vi "Booean to T-F string.vi"(4 "Boolean iin":bool) -> (1 "T/F String":string)   [LabVIEW 2009, in "Strings Lib.lvlib"]
doc: "Converts a boolean to 'T' or 'F' String. Used for shortened notation file io."
uses:
  Strings Lib.lvlib
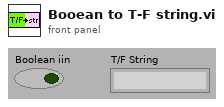
[diagram p1: front panel]
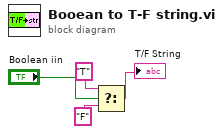
[diagram p0: block diagram]
diagram:
  n1 = Select(t="T", s="Boolean iin", f="F") -> (s? t:f=→"T/F String":string)
